vi "Get Database Item.vi"(8 "error in (no error)":errorcluster, 10 "id":u32, 11 "eLab in":refnum<class "PL eLabFTW Client.lvclass">) -> (0 "error out":errorcluster, 2 "database item":T1 {"steps"."finish datetime" format="%<%X\n%x>T"; "steps"."deadline datetime" format="%<%X\n%x>T"; "files"."creation datetime" format="%<%X\n%x>T"; "last change"."datetime" format="%<%X\n%x>T"; "start datetime" format="%<%X\n%x>T"; "last comment"."datetime" format="%<%X\n%x>T"; "lock"."datetime" format="%<%X\n%x>T"}, 3 "eLab out":refnum<class "PL eLabFTW Client.lvclass">)   [LabVIEW 2015, in "PL eLabFTW Client.lvclass"]
doc: "Gets database item with the specified id."
uses:
  PL eLabFTW Client.lvclass
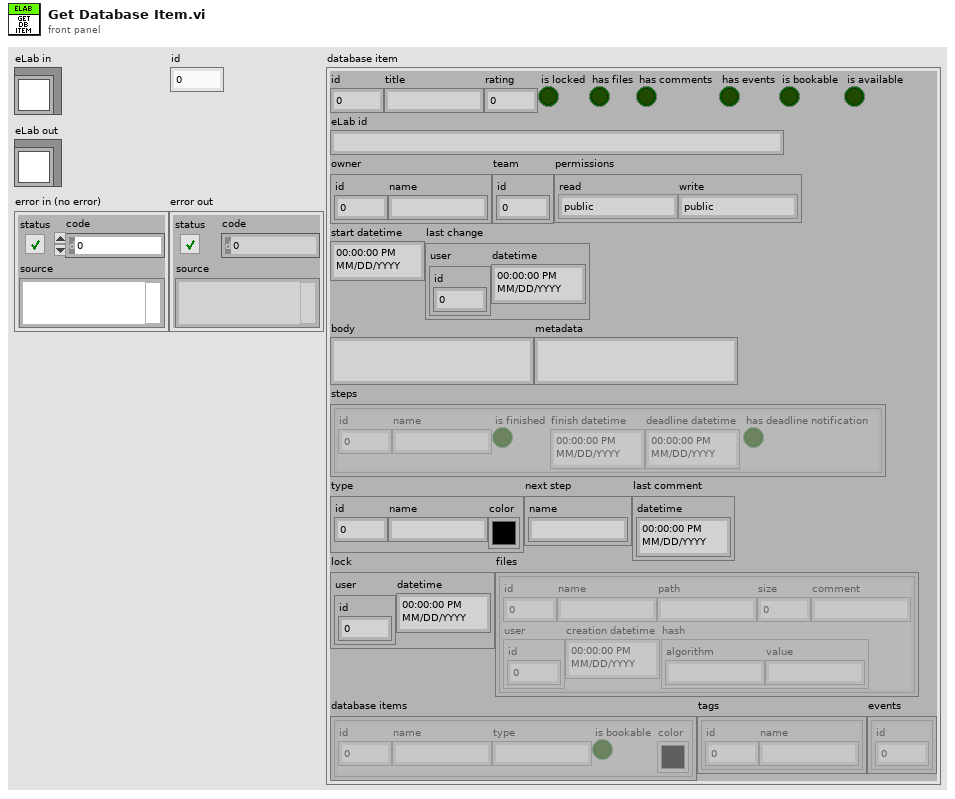
[diagram p1: front panel]
types:
  T1 = cluster{"id":u32, "title":string, "rating":u32, "is locked":bool, "has files":bool, "has comments":bool, "has events":bool, "is bookable":bool, "is available":bool, "eLab id":string, "owner":cluster{"id":u32, "name":string}, "team":cluster{"id":u32}, "permissions":cluster{"read":enum16{"public", "organization", "team", "owner and admins", "owner"}, "write":enum16{"public", "organization", "team", "owner and admins", "owner"}}, "start datetime":timestamp, "last change":cluster{"user":cluster{"id":u32}, "datetime":timestamp}, "body":string, "metadata":string, "steps":cluster{"id":u32, "name":string, "is finished":bool, "finish datetime":timestamp, "deadline datetime":timestamp, "has deadline notification":bool}[], "type":cluster{"id":u32, "name":string, "color":u32}, "next step":cluster{"name":string}, "last comment":cluster{"datetime":timestamp}, "lock":cluster{"user":cluster{"id":u32}, "datetime":timestamp}, "files":cluster{"id":u32, "name":string, "path":string, "size":u32, "comment":string, "user":cluster{"id":u32}, "creation datetime":timestamp, "hash":cluster{"algorithm":string, "value":string}}[], "database items":cluster{"id":u32, "name":string, "type":string, "is bookable":bool, "color":u32}[], "tags":cluster{"id":u32, "name":string}[], "events":cluster{"id":u32}[]}
  T2 = cluster{"id":string, "team":string, "title":string, "date":string, "body":string, "rating":string, "category":string, "locked":string, "lockedby":string, "lockedwhen":string, "userid":string, "canread":string, "canwrite":string, "available":string, "lastchange":string, "elabid":string, "metadata":string, "lastchangeby":string, "state":string, "is_bound":string, "events_item_id":string, "events_id":string, "up_item_id":string, "has_attachment":string, "next_step":string, "category_id":string, "color":string, "fullname":string, "recent_comment":string, "has_comment":string, "bookable":string, "tags":string, "tags_id":string, "uploads":cluster{"id":string, "real_name":string, "long_name":string, "comment":string, "item_id":string, "userid":string, "type":string, "created_at":string, "hash":string, "hash_algorithm":string, "storage":string, "filesize":string, "state":string}[], "links":cluster{"itemid":string, "title":string, "name":string, "bookable":string, "color":string}[], "steps":cluster{"id":string, "item_id":string, "body":string, "ordering":string, "finished":string, "finished_time":string, "deadline":string, "deadline_notif":string}[]}
  T3 = cluster{"id":i32, "team":i32, "title":i32, "date":i32, "body":i32, "rating":i32, "category":i32, "locked":i32, "lockedby":i32, "lockedwhen":i32, "userid":i32, "canread":i32, "canwrite":i32, "available":i32, "lastchange":i32, "elabid":i32, "metadata":i32, "lastchangeby":i32, "state":i32, "is_bound":i32, "events_item_id":i32, "events_id":i32, "up_item_id":i32, "has_attachment":i32, "next_step":i32, "category_id":i32, "color":i32, "fullname":i32, "recent_comment":i32, "has_comment":i32, "bookable":i32, "tags":i32, "tags_id":i32, "uploads":cluster{"id":i32, "real_name":i32, "long_name":i32, "comment":i32, "item_id":i32, "userid":i32, "type":i32, "created_at":i32, "hash":i32, "hash_algorithm":i32, "storage":i32, "filesize":i32, "state":i32}[], "links":cluster{"itemid":i32, "title":i32, "name":i32, "bookable":i32, "color":i32}[], "steps":cluster{"id":i32, "item_id":i32, "body":i32, "ordering":i32, "finished":i32, "finished_time":i32, "deadline":i32, "deadline_notif":i32}[]}
  T4 = cluster{"id":string, "item_id":string, "body":string, "ordering":string, "finished":string, "finished_time":string, "deadline":string, "deadline_notif":string}[]
  T5 = cluster{"id":string, "real_name":string, "long_name":string, "comment":string, "item_id":string, "userid":string, "type":string, "created_at":string, "hash":string, "hash_algorithm":string, "storage":string, "filesize":string, "state":string}[]
  T6 = cluster{"itemid":string, "title":string, "name":string, "bookable":string, "color":string}[]
  T7 = cluster{"id":bool, "team":bool, "title":bool, "date":bool, "body":bool, "rating":bool, "category":bool, "locked":bool, "lockedby":bool, "lockedwhen":bool, "userid":bool, "canread":bool, "canwrite":bool, "available":bool, "lastchange":bool, "elabid":bool, "metadata":bool, "lastchangeby":bool, "state":bool, "is_bound":bool, "events_item_id":bool, "events_id":bool, "up_item_id":bool, "has_attachment":bool, "next_step":bool, "category_id":bool, "color":bool, "fullname":bool, "recent_comment":bool, "has_comment":bool, "bookable":bool, "tags":bool, "tags_id":bool, "uploads":cluster{"id":bool, "real_name":bool, "long_name":bool, "comment":bool, "item_id":bool, "userid":bool, "type":bool, "created_at":bool, "hash":bool, "hash_algorithm":bool, "storage":bool, "filesize":bool, "state":bool}[], "links":cluster{"itemid":bool, "title":bool, "name":bool, "bookable":bool, "color":bool}[], "steps":cluster{"id":bool, "item_id":bool, "body":bool, "ordering":bool, "finished":bool, "finished_time":bool, "deadline":bool, "deadline_notif":bool}[]}
  T8 = cluster{"id":i32, "item_id":i32, "body":i32, "ordering":i32, "finished":i32, "finished_time":i32, "deadline":i32, "deadline_notif":i32}
  T9 = cluster{"id":bool, "item_id":bool, "body":bool, "ordering":bool, "finished":bool, "finished_time":bool, "deadline":bool, "deadline_notif":bool}
  T10 = cluster{"id":u32, "name":string, "is finished":bool, "finish datetime":timestamp, "deadline datetime":timestamp, "has deadline notification":bool}
  T11 = cluster{"id":i32, "real_name":i32, "long_name":i32, "comment":i32, "item_id":i32, "userid":i32, "type":i32, "created_at":i32, "hash":i32, "hash_algorithm":i32, "storage":i32, "filesize":i32, "state":i32}
  T12 = cluster{"id":u32, "name":string, "path":string, "size":u32, "comment":string, "user":cluster{"id":u32}, "creation datetime":timestamp, "hash":cluster{"algorithm":string, "value":string}}
  T13 = cluster{"itemid":i32, "title":i32, "name":i32, "bookable":i32, "color":i32}
  T14 = cluster{"itemid":bool, "title":bool, "name":bool, "bookable":bool, "color":bool}
  T15 = cluster{"id":u32, "name":string, "type":string, "is bookable":bool, "color":u32}
  T16 = enum16{"public", "organization", "team", "owner and admins", "owner"}
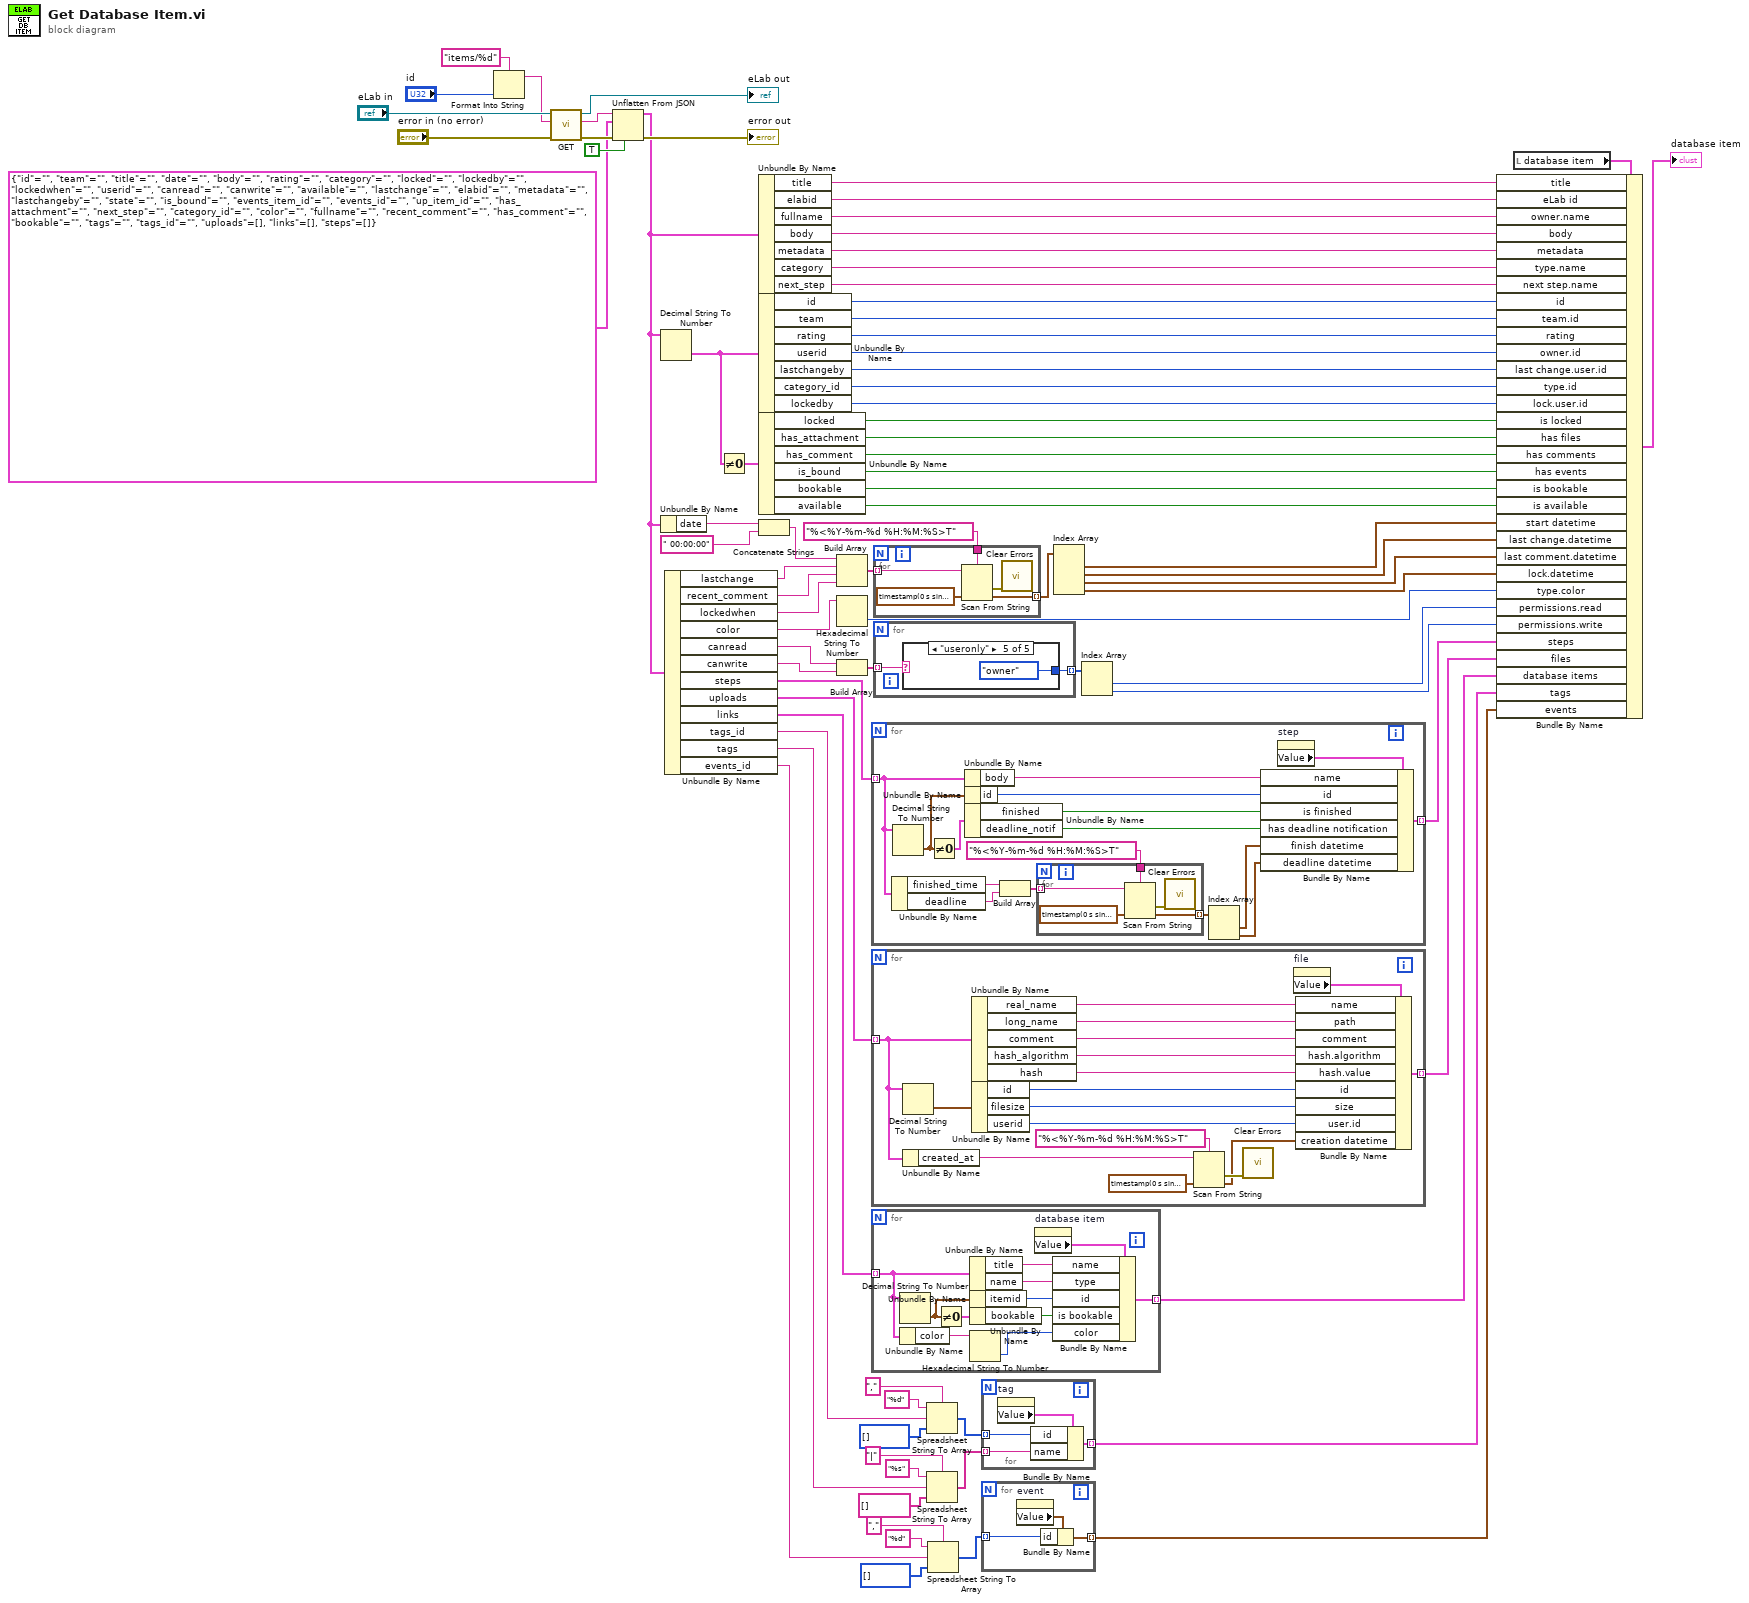
[diagram p0: block diagram]
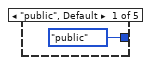
[diagram p2: hidden frame]
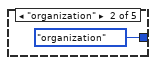
[diagram p3: hidden frame]
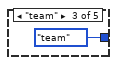
[diagram p4: hidden frame]
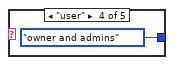
[diagram p5: hidden frame]
diagram:
  n1 = Format Into String(format string="items/%d", "id") -> (resulting string=w73:string)  [unwired: 2 in, 1 out]
  n2 = call "GET.vi"("error in (no error)"="error in (no error)", "relative URL"=w73, "eLab in"="eLab in") -> ("error out"=w77:errorcluster, "response body"=w1:string, "eLab out"=→"eLab out":refnum<class "PL eLabFTW Client.lvclass">)  [unwired: 6 in]
  n3 = Unflatten From JSON(JSON string=w1, type and defaults=T2 {"id"="", "team"="", "title"="", "date"="", "body"="", "rating"="", "category"="", "locked"="", "lockedby"="", "lockedwhen"="", "userid"="", "canread"="", "canwrite"="", "available"="", "lastchange"="", "elabid"="", "metadata"="", "lastchangeby"="", "state"="", "is_bound"="", "events_item_id"="", "events_id"="", "up_item_id"="", "has_attachment"="", "next_step"="", "category_id"="", "color"="", "fullname"="", "recent_comment"="", "has_comment"="", "bookable"="", "tags"="", "tags_id"="", "uploads"=[], "links"=[], "steps"=[]}, default null elements? (F)=TRUE, error in (no error)=w77) -> (value=w29:T2, error out=→"error out":errorcluster)  [unwired: 3 in]
  n4 = Decimal String To Number(string=w29) -> (number=w62:T3)  [unwired: 2 in, 1 out]
  n5 = Unbundle By Name(w29) -> ("date"=w41:string)
  n6 = Unbundle By Name(w29) -> ("lastchange"=w56:string, "recent_comment"=w57:string, "lockedwhen"=w36:string, "color"=w51:string, "canread"=w49:string, "canwrite"=w48:string, "steps"=w27:T4, "uploads"=w25:T5, "links"=w23:T6, "tags_id"=w14:string, "tags"=w13:string, "events_id"=w11:string)
  n7 = Not Equal To 0?(x=w62) -> (x != 0?=w61:T7)
  n8 = Unbundle By Name(w29) -> ("title"=w70:string, "elabid"=w37:string, "fullname"=w69:string, "body"=w38:string, "metadata"=w34:string, "category"=w68:string, "next_step"=w67:string)
  n9 = Unbundle By Name(w62) -> ("id"=w66:i32, "team"=w4:i32, "rating"=w65:i32, "userid"=w64:i32, "lastchangeby"=w30:i32, "category_id"=w63:i32, "lockedby"=w33:i32)
  n10 = Unbundle By Name(w61) -> ("locked"=w60:bool, "has_attachment"=w59:bool, "has_comment"=w58:bool, "is_bound"=w5:bool, "bookable"=w3:bool, "available"=w2:bool)
  n11 = Concatenate Strings(w41, " 00:00:00" ("string")) -> (w40:string)
  n12 = Build Array(w40, w56, w57, w36) -> (w55:string[])
  n13 = Hexadecimal String To Number(string=w51) -> (number=w50:u32)  [unwired: 2 in, 1 out]
  n14 = Build Array(w49, w48) -> (w47:string[])
  n15 = for {
    tunnel: [w95] -> w28 mode=indexing
    tunnel: w27 -> [w88] mode=indexing
    n16 = Unbundle By Name(w88) -> ("finished_time"=w86:string, "deadline"=w85:string)
    n17 = Decimal String To Number(string=w88) -> (number=w92:T8)  [unwired: 2 in, 1 out]
    n18 = Not Equal To 0?(x=w92) -> (x != 0?=w91:T9)
    n19 = Unbundle By Name(w88) -> ("body"=w94:string)
    n20 = Unbundle By Name(w92) -> ("id"=w93:i32)
    n21 = Unbundle By Name(w91) -> ("finished"=w90:bool, "deadline_notif"=w89:bool)
    n22 = Build Array(w86, w85) -> (w84:string[])
    n23 = for {
      tunnel: w84 -> [w99] mode=indexing
      tunnel: [w98] -> w83 mode=indexing
      tunnel: "%<%Y-%m-%d %H:%M:%S>T" ("format string") -> [w97]
      n24 = Scan From String(format string=w97, input string=w99, default 1=timestamp(0 s since 1904-01-01) ("from")) -> (error out=w101:errorcluster, output 1=w98:timestamp)  [unwired: 2 in, 2 out]
      n25 = call <vilib>:"Clear Errors.vi"("error in (no error)"=w101) -> ()  [unwired: 5 in, 2 out]
    }
    n26 = Index Array(array=w83) -> (element #1=w82:timestamp, element #2=w81:timestamp)  [unwired: 2 in]
    n27 = property on="step" class="Clust (strict)"() -> ("Value"=w96:T10)  [unwired: 2 in, 2 out]
    n28 = Bundle By Name(cluster=w96, "name"=w94, "id"=w93, "is finished"=w90, "has deadline notification"=w89, "finish datetime"=w82, "deadline datetime"=w81) -> (w95:T10)
  }
  n29 = for {
    tunnel: [w117] -> w26 mode=indexing
    tunnel: w25 -> [w103] mode=indexing
    n30 = Decimal String To Number(string=w103) -> (number=w111:T11)  [unwired: 2 in, 1 out]
    n31 = Unbundle By Name(w103) -> ("created_at"=w104:string)
    n32 = Unbundle By Name(w103) -> ("real_name"=w116:string, "long_name"=w115:string, "comment"=w114:string, "hash_algorithm"=w113:string, "hash"=w112:string)
    n33 = Unbundle By Name(w111) -> ("id"=w108:i32, "filesize"=w109:i32, "userid"=w110:i32)
    n34 = Scan From String(format string="%<%Y-%m-%d %H:%M:%S>T", input string=w104, default 1=timestamp(0 s since 1904-01-01) ("from")) -> (error out=w106:errorcluster, output 1=w102:timestamp)  [unwired: 2 in, 2 out]
    n35 = call <vilib>:"Clear Errors.vi"("error in (no error)"=w106) -> ()  [unwired: 5 in, 2 out]
    n36 = property on="file" class="Clust (strict)"() -> ("Value"=w118:T12)  [unwired: 2 in, 2 out]
    n37 = Bundle By Name(cluster=w118, "name"=w116, "path"=w115, "comment"=w114, "hash.algorithm"=w113, "hash.value"=w112, "id"=w108, "size"=w109, "user.id"=w110, "creation datetime"=w102) -> (w117:T12)
  }
  n38 = for {
    tunnel: [w128] -> w24 mode=indexing
    tunnel: w23 -> [w123] mode=indexing
    n39 = Decimal String To Number(string=w123) -> (number=w126:T13)  [unwired: 2 in, 1 out]
    n40 = Unbundle By Name(w123) -> ("color"=w120:string)
    n41 = Not Equal To 0?(x=w126) -> (x != 0?=w127:T14)
    n42 = Unbundle By Name(w123) -> ("title"=w125:string, "name"=w124:string)
    n43 = Unbundle By Name(w126) -> ("itemid"=w122:i32)
    n44 = Unbundle By Name(w127) -> ("bookable"=w121:bool)
    n45 = Hexadecimal String To Number(string=w120) -> (number=w119:u32)  [unwired: 2 in, 1 out]
    n46 = property on="database item" class="Clust (strict)"() -> ("Value"=w129:T15)  [unwired: 2 in, 2 out]
    n47 = Bundle By Name(cluster=w129, "name"=w125, "type"=w124, "id"=w122, "is bookable"=w121, "color"=w119) -> (w128:T15)
  }
  n48 = for {
    tunnel: w55 -> [w132] mode=indexing
    tunnel: [w131] -> w54 mode=indexing
    tunnel: "%<%Y-%m-%d %H:%M:%S>T" ("format string") -> [w130]
    n49 = Scan From String(format string=w130, input string=w132, default 1=timestamp(0 s since 1904-01-01) ("from")) -> (error out=w134:errorcluster, output 1=w131:timestamp)  [unwired: 2 in, 2 out]
    n50 = call <vilib>:"Clear Errors.vi"("error in (no error)"=w134) -> ()  [unwired: 5 in, 2 out]
  }
  n51 = for {
    tunnel: w47 -> [w136] mode=indexing
    tunnel: [w135] -> w46 mode=indexing
    n52 = case shown="\"useronly\"" w136 {
      tunnel: [T16."public" ("permissions.read") T16."organization" ("permissions.read") T16."team" ("permissions.read") T16."owner and admins" ("permissions.read") T16."owner" ("permissions.read")] -> w135
      frame "public", Default {
      }
      frame "organization" {
      }
      frame "team" {
      }
      frame "user" {
      }
      frame "useronly" {
      }
    }
  }
  n53 = Spreadsheet String To Array(delimiter (Tab)=",", format string="%d", spreadsheet string=w14, array type (2D Dbl)=u32[] []) -> (array=w10:u32[])
  n54 = Spreadsheet String To Array(delimiter (Tab)="|", format string="%s", spreadsheet string=w13, array type (2D Dbl)=string[] []) -> (array=w9:string[])
  n55 = Spreadsheet String To Array(delimiter (Tab)=",", format string="%d", spreadsheet string=w11, array type (2D Dbl)=u32[] []) -> (array=w7:u32[])
  n56 = for {
    tunnel: [w144] -> w8 mode=indexing
    tunnel: w10 -> [w143] mode=indexing
    tunnel: w9 -> [w142] mode=indexing
    n57 = property on="tag" class="Clust (strict)"() -> ("Value"=w145:cluster{"id":u32, "name":string})  [unwired: 2 in, 2 out]
    n58 = Bundle By Name(cluster=w145, "id"=w143, "name"=w142) -> (w144:cluster{"id":u32, "name":string})
  }
  n59 = for {
    tunnel: [w147] -> w6 mode=indexing
    tunnel: w7 -> [w146] mode=indexing
    n60 = property on="event" class="Clust (strict)"() -> ("Value"=w148:cluster{"id":u32})  [unwired: 2 in, 2 out]
    n61 = Bundle By Name(cluster=w148, "id"=w146) -> (w147:cluster{"id":u32})
  }
  n62 = Index Array(array=w54) -> (element #1=w42:timestamp, element #2=w53:timestamp, element #3=w52:timestamp, element #4=w35:timestamp)  [unwired: 4 in]
  n63 = Index Array(array=w46) -> (element #1=w45:T16, element #2=w44:T16)  [unwired: 2 in]
  n64 = local read "database item"() -> (w32:T1)
  n65 = Bundle By Name(cluster=w32, "title"=w70, "eLab id"=w37, "owner.name"=w69, "body"=w38, "metadata"=w34, "type.name"=w68, "next step.name"=w67, "id"=w66, "team.id"=w4, "rating"=w65, "owner.id"=w64, "last change.user.id"=w30, "type.id"=w63, "lock.user.id"=w33, "is locked"=w60, "has files"=w59, "has comments"=w58, "has events"=w5, "is bookable"=w3, "is available"=w2, "start datetime"=w42, "last change.datetime"=w53, "last comment.datetime"=w52, "lock.datetime"=w35, "type.color"=w50, "permissions.read"=w45, "permissions.write"=w44, "steps"=w28, "files"=w26, "database items"=w24, "tags"=w8, "events"=w6) -> (→"database item":T1)
